vi "DefaultFromINI.vi"(8 "error in (no error)":errorcluster, 11 "ChromaAcLoad":refnum<class "ChromaAcLoad.lvclass">) -> (0 "error out":errorcluster, 3 "ChromaAcLoad":refnum<class "ChromaAcLoad.lvclass">)   [LabVIEW 2018, in "AcPwrPlugins.lvlib" / "ChromaAcLoad.lvclass"]
doc: "This VI reads the properties from the INI file and puts them into the LabVIEW class for further use."
uses:
  ChromaAcLoad.lvclass
  C:/Program Files (x86)/National Instruments/LabVIEW 2018/user.lib/NIST/BaseClasses/BasePlugin_class/BasePlugin.lvclass
  C:/Users/Public/Projects/ICDAS/NistPluggableModules/AcPwr/AcPwrPlugins/AcPwrBaseClass/AcPwrBase.lvclass
  TypeDefs/Device(s)Settings.ctl
  TypeDefs/Measurements.ctl
  TypeDefs/MeasurementType.ctl
  <userlib>/NIST/BaseClasses/BasePlugin_class/BasePlugin.lvclass/BasePlugin.ctl
  <userlib>/NIST/BaseClasses/BasePlugin_class/Accessors/Read PluginIniFilePath.vi
  AcPwrBaseClass/AcPwrBase.lvclass
  <vilib>/Utility/config.llb/NI_LVConfig.lvlib
  TestClass/Test.lvclass
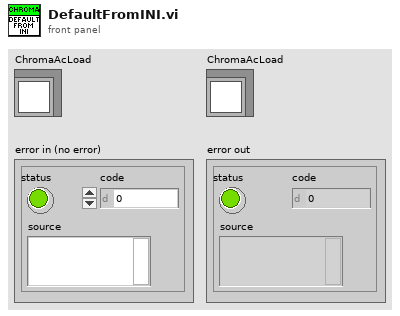
[diagram p1: front panel]
types:
  T1 = typedef "AcPwrPlugins.lvlib/ChromaAcLoad.lvclass/Measurements.ctl" = cluster{"Handle":string, "Name":string, "Enabled":bool, "Measurement Value":dbl, "Hold Peak Current Measurement":bool, "btnMeasFetch":bool, "ProtectionStatusString":string, "Measurement Type":T2}[]
  T2 = typedef "AcPwrPlugins.lvlib/ChromaAcLoad.lvclass/MeasurementType.ctl" = enum16{"Voltage (Vrms or V)", "Current (Arms or A)", "Power (W)", "Peak Voltage (V)", "Peak Current (A)", "Peak Power (W)", "Frequency (Hz)", "Resistance (Ohms)", "Voltage Overshoot (V)", "Positive Peak Current (A)", "Voltage Undershoot (V)", "Negative Peak Current (A)", "Apparent Power (VA)", "Reacitive Power (VAR)", "Voltage THD", "Power Factor", "Current's Crest Factor"}
  T3 = typedef "AcPwrPlugins.lvlib/ChromaAcLoad.lvclass/Device(s)Settings.ctl" = cluster{"Configuration Mode":enum16{"Constant Voltage (DC)", "Constant Power (DC)", "Constant Power (AC)", "Constant Current (DC)", "Constant Current (AC)", "Constant Resistance (DC)", "Constant Resistance (AC)", "Rectified Mode (DC)", "Inrush (AC)", "RLC CP (AC)", "RLC (AC)"}, "Phases":cluster{"Handle":string, "Name":string, "Phase Select":i32, "Instrument Options":string, "id query (T)":bool, "reset device (T)":bool, "Load Short Circuited":bool, "Line Synchronization":bool, "Load Current (A/Arms)":dbl, "Load Voltage (V/Vrms)":dbl, "Load Power (W)":dbl, "Load Resistance (Ohms)":dbl, "Load Current Peak Limit (A)":dbl, "Load Current Limit (A/Arms)":dbl, "Load Power Limit (W)":dbl, "Synch Frequency (Hz)":dbl, "Priority":enum16{"CF Only", "PF Only", "Both (CF)", "Both (PF)"}, "Crest Factor":dbl, "Power Factor":dbl, "Slew Rate":cluster{"Rise Slew Rate (A/ms)":i32, "Fall Slew Rate (A/ms)":i32}, "LC/RLC Mode":cluster{"Capacitance (uF)":i32, "Inductance (uH)":i32, "Series Resistance (Ohm)":dbl, "Parallel Resistance (Ohm)":dbl}, "Timing":cluster{"TimingOn":enum16{""}, "Hours":u32, "Minutes":u32, "Seconds":dbl, "CutoffVoltage":dbl}, "Connected":bool}[], "MeasName":string}
  T4 = typedef "NI_LVConfig.lvlib/Config Data RefNum.ctl" = refnum<k1>
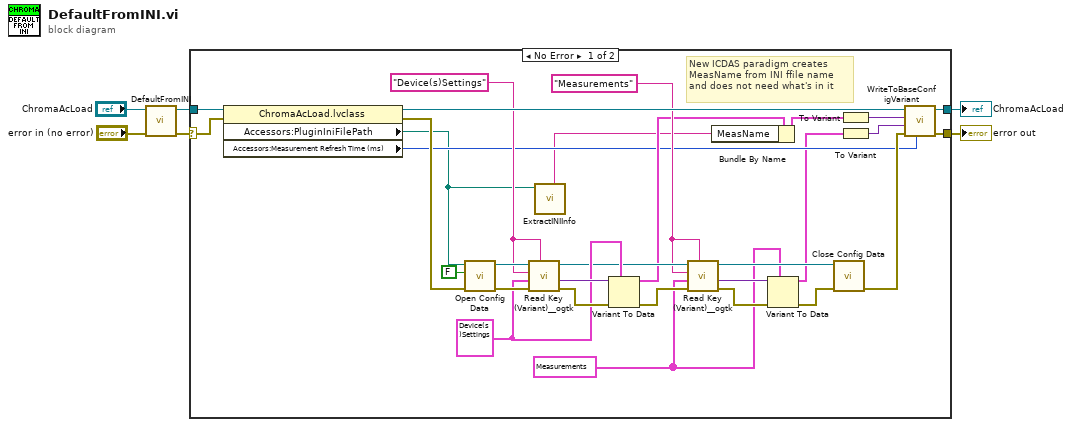
[diagram p0: block diagram]
diagram:
  n1 = call-parent "DefaultFromINI.vi"("error in (no error)"="error in (no error)", "AcPwrBase"="ChromaAcLoad") -> ("error out"=w4:errorcluster, "AcPwrBase"=w3:refnum<class "ChromaAcLoad.lvclass">)  [unwired: 8 in]
  n2 = case shown="No Error" w4 {
    selector: w4 -> [w28 w37]
    tunnel: w3 -> [w36 w38]
    tunnel: [w15 w38] -> w2
    tunnel: [w14 w37] -> w1
    frame No Error {
      w17 = "Measurements" ("section")
      w18 = T1 [{"Handle"="", "Name"="", "Enabled"=FALSE, "Measurement Value"=0.0, "Hold Peak Current Measurement"=FALSE, "btnMeasFetch"=TRUE, "ProtectionStatusString"="", "Measurement Type"=enum."Voltage (Vrms or V)"}] ("Measurements")
      w25 = T3 {"Configuration Mode"=enum."Constant Voltage (DC)", "Phases"=[], "MeasName"=""} ("Device Properties")
      w29 = "Device(s)Settings" ("section")
      # "New ICDAS paradigm creates\nMeasName from INI ffile name\nand does not need what's in it"
      n3 = property class="ChromaAcLoad.lvclass"(reference=w36, error in=w28) -> (reference out=w30:refnum<class "ChromaAcLoad.lvclass">, error out=w27:errorcluster, "Accessors:PluginIniFilePath"=w8:path, "Accessors:Measurement Refresh Time (ms)"=w12:u32)
      n4 = call <vilib>:"Open Config Data.vi"("error in (no error)"=w27, "create file if necessary (T)"=FALSE, "configuration file path"=w8) -> ("error out"=w33:errorcluster, "refnum"=w34:T4)  [unwired: 6 in, 1 out]
      n5 = call <userlib>:"Read Key (Variant)__ogtk.vi"("section"=w29, "error in (no error)"=w33, "type"=w25, "key (optional)"=w29, "refnum"=w34) -> ("error out"=w31:errorcluster, "key-value"=w32:variant, "refnum out"=w22:T4)  [unwired: 3 in, 1 out]
      n6 = call "ExtractINIInfo.vi"("INI File Path"=w8) -> ("Module.Class.INI File Name"=w7:string)  [unwired: 4 in, 6 out]
      n7 = Variant To Data(error in=w31, type=w25, Variant=w32) -> (data=w13:T3, error out=w19:errorcluster)
      n8 = call <userlib>:"Read Key (Variant)__ogtk.vi"("section"=w17, "error in (no error)"=w19, "type"=w18, "key (optional)"=w17, "refnum"=w22) -> ("error out"=w24:errorcluster, "key-value"=w23:variant, "refnum out"=w21:T4)  [unwired: 3 in, 1 out]
      n9 = Bundle By Name(cluster=w13, "MeasName"=w7) -> (w9:T3)
      n10 = Variant To Data(error in=w24, type=w18, Variant=w23) -> (data=w11:T1, error out=w20:errorcluster)
      n11 = call <vilib>:"Close Config Data.vi"("error in (no error)"=w20, "refnum"=w21) -> ("error out"=w26:errorcluster)  [unwired: 8 in, 1 out]
      n12 = To Variant(anything=w9) -> (Variant=w16:variant)
      n13 = To Variant(anything=w11) -> (Variant=w10:variant)
      n14 = call "WriteToBaseConfigVariant.vi"("Measurement Refresh Time (ms)"=w12, "error in (no error)"=w26, "Meas"=w10, "Config"=w16, "ChromaAcLoad in"=w30) -> ("error out"=w14:errorcluster, "ChromaAcLoad out"=w15:refnum<class "ChromaAcLoad.lvclass">)  [unwired: 5 in]
    }
    frame Error {
    }
  }
  "error out" <- w1
  "ChromaAcLoad" <- w2
